vi "TDT-Sort Events.vi"(8 "Tosca Markers":dbl[][](array[numeric]), 9 "Artifacts":dbl[][](array[numeric]), 10 "Spikes":dbl[][](array[numeric]), 11 "Ticks":dbl[][](array[numeric])) -> (3 "Sorted events":dbl[][](array[numeric]))   [LabVIEW 2020]
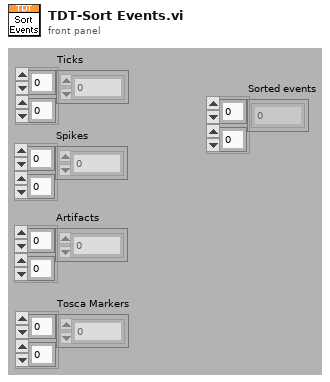
[diagram p1: front panel]
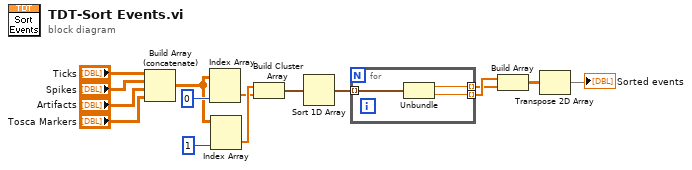
[diagram p0: block diagram]
diagram:
  n1 = Build Array (concatenate)("Ticks", "Spikes", "Artifacts", "Tosca Markers") -> (w13:dbl[][])
  n2 = Index Array(array=w13, index (col)=0 ("disabled index (col)")) -> (element=w11:dbl[])  [unwired: 1 in]
  n3 = Index Array(array=w13, index (col)=1) -> (element=w12:dbl[])  [unwired: 1 in]
  n4 = Build Cluster Array(w12, w11) -> (w10:cluster{"Numeric":dbl, "Numeric":dbl}[])
  n5 = Sort 1D Array(array=w10) -> (sorted array=w4:cluster{"Numeric":dbl, "Numeric":dbl}[])
  n6 = for {
    tunnel: w4 -> [w18] mode=indexing
    tunnel: [w17] -> w9 mode=indexing
    tunnel: [w16] -> w8 mode=indexing
    n7 = Unbundle(w18) -> ("Numeric"=w16:dbl, "Numeric"=w17:dbl)
  }
  n8 = Build Array(w9, w8) -> (w7:dbl[][])
  n9 = Transpose 2D Array(2D array=w7) -> (transposed array=→"Sorted events":dbl[][])
